vi "Collect Map Entries.vi"(8 "error in (no error)":errorcluster, 11 "LV-Protoc in":refnum<class "LV-Protoc.lvclass">) -> (0 "error out":errorcluster, 2 "Map Fields":T1[](array[typedef]), 3 "LV-Protoc out":refnum<class "LV-Protoc.lvclass">)   [LabVIEW 2020, in "LV-Protoc.lvlib" / "LV-Protoc.lvclass"]
uses:
  LV-Protoc.lvclass
  Map Definition.ctl
  LV-Proto/Field.ctl
  LV-Proto/Type.ctl
  LV-Proto/Proto Type.ctl
  LV-Protoc.lvclass/LV-Protoc.ctl
  LV-Proto/LV-Proto.lvlib
  LV-Protoc.lvlib
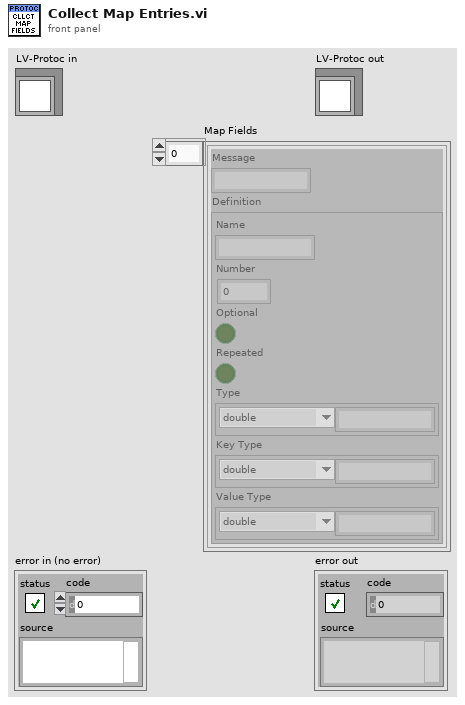
[diagram p1: front panel]
types:
  T1 = typedef "LV-Protoc.lvlib/Map Definition.ctl" = cluster{"Message":string, "Definition":T2}
  T2 = typedef "LV-Proto.lvlib/Field.ctl" = cluster{"Name":string, "Number":u32, "Optional":bool, "Repeated":bool, "Type":T3, "Key Type":T3, "Value Type":T3}
  T3 = typedef "LV-Proto.lvlib/Type.ctl" = cluster{"Type":T4, "Subtype":string}
  T4 = typedef "LV-Proto.lvlib/Proto Type.ctl" = enum16{"UNKNOWN", "double", "float", "int32", "int64", "uint32", "uint64", "sint32", "sint64", "fixed32", "fixed64", "sfixed32", "sfixed64", "bool", "string", "bytes", "enum", "map", "message"}
  T5 = typedef "LV-Proto.lvlib/Message.ctl" = cluster{"Name":string, "Fields":T2[], "Reserved Numbers":u32[], "Reserved Names":string[]}
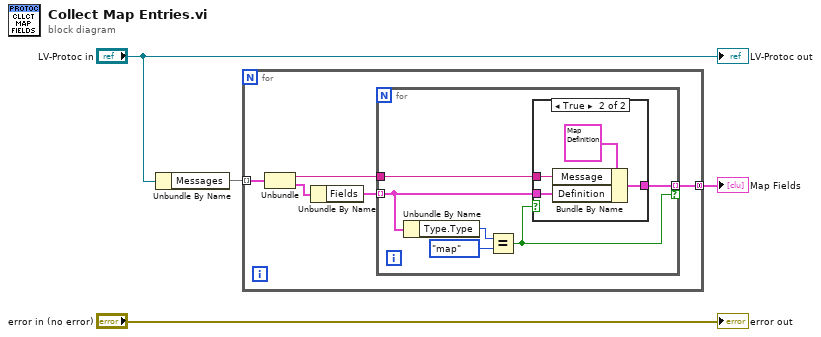
[diagram p0: block diagram]
diagram:
  n1 = Unbundle By Name("LV-Protoc in") -> ("Messages"=w4:map{string, T5})
  n2 = for {
    tunnel: w4 -> [w9] mode=indexing
    tunnel: [w5] -> w3 mode=concatenating
    n3 = Unbundle(w9) -> ("Name"=w6:string, "Message"=w8:T5)
    n4 = Unbundle By Name(w8) -> ("Fields"=w7:T2[])
    n5 = for {
      tunnel: w7 -> [w13] mode=indexing
      tunnel: w6 -> [w12]
      tunnel: [w11] -> w5 mode=indexing if=w10
      n6 = Unbundle By Name(w13) -> ("Type.Type"=w15:T4)
      n7 = Equal?(x=w15, y=Proto_Type."map") -> (x = y?=w10:bool)
      n8 = case shown="True" w10 {
        tunnel: w13 -> [_ w18]
        tunnel: w12 -> [_ w17]
        tunnel: [_ w16] -> w11
        frame False {
        }
        frame True {
          n9 = Bundle By Name(cluster=T1 {"Message"="", "Definition"={"Name"="", "Number"=0, "Optional"=FALSE, "Repeated"=FALSE, "Type"={"Type"=enum."double", "Subtype"=""}, "Key Type"={"Type"=enum."double", "Subtype"=""}, "Value Type"={"Type"=enum."double", "Subtype"=""}}} ("Map Definition"), "Message"=w17, "Definition"=w18) -> (w16:T1)
        }
      }
    }
  }
  "Map Fields" <- w3
  "error out" <- "error in (no error)"
  "LV-Protoc out" <- "LV-Protoc in"
